vi "Puntje 2 implementeren kladversie.vi"() -> ()   [LabVIEW 2019]
panel:
  in  "Slide 2":dbl(slide) scale=0.0..10.0
  in  "Slide":dbl(slide) scale=0.0..10.0
  out "linkermotor":dbl(knob) scale=0.0..10.0
  out "rechtermotor":dbl(knob) scale=0.0..10.0
  in  "Array":dbl[](array[numeric])
  # "5 : neemt volledig WITTE regio waar"
  # "0 : neemt volledige ZWARTE regio waar"
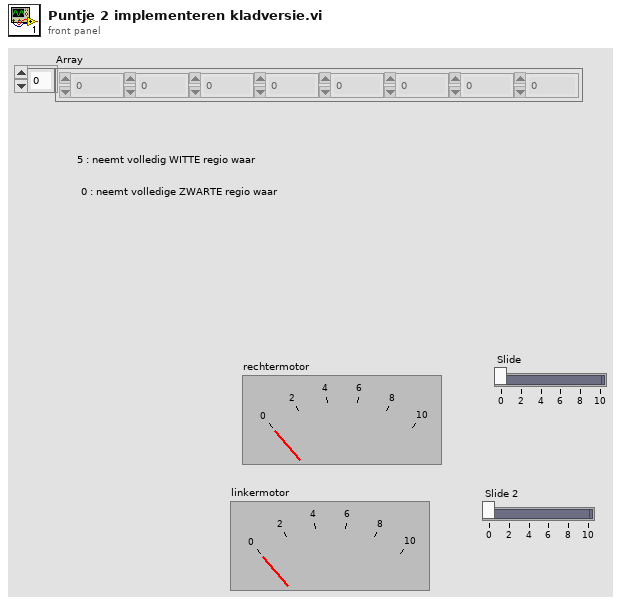
[diagram p1: front panel]
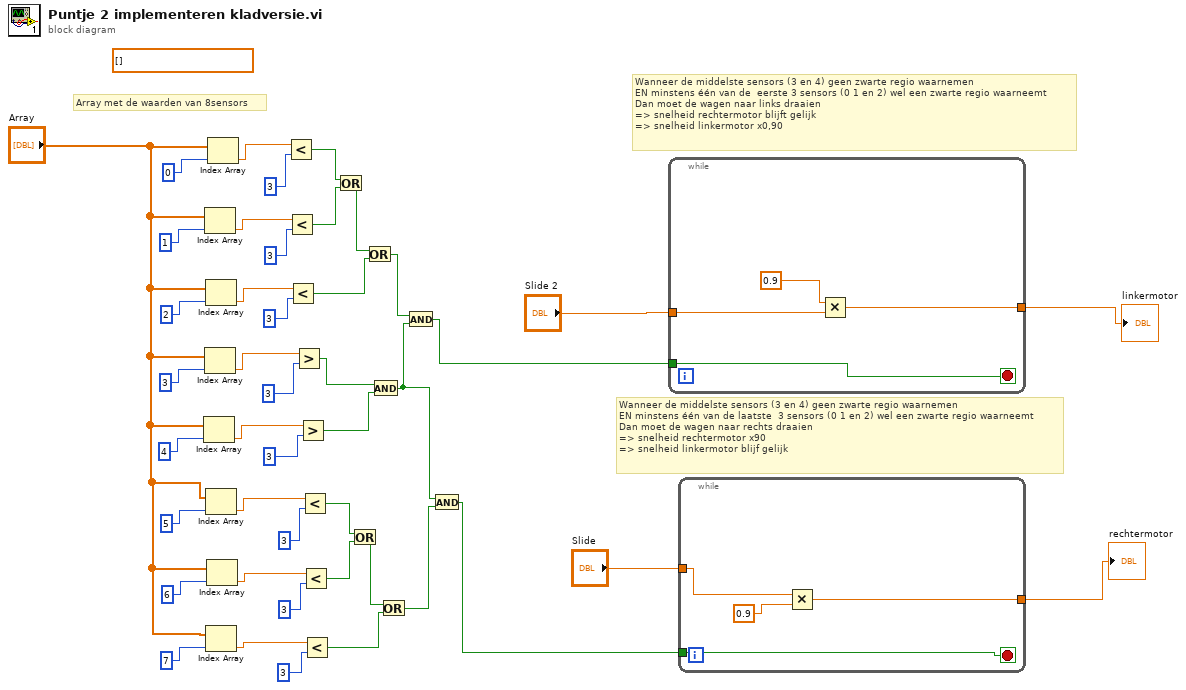
[diagram p0: block diagram]
diagram:
  (unwired) dbl[] []
  # "Wanneer de middelste sensors (3 en 4) geen zwarte regio waarnemen\nEN minstens één van de laatste  3 sensors (0 1 en 2) wel een zwarte regio waarneemt \nDan moet de wagen naar rechts draaien \n=> snelheid rechtermotor x90\n=> snelheid linkermotor blijf gelijk"
  # "Wanneer de middelste sensors (3 en 4) geen zwarte regio waarnemen\nEN minstens één van de  eerste 3 sensors (0 1 en 2) wel een zwarte regio waarneemt \nDan moet de wagen naar links draaien \n=> snelheid rechtermotor blijft gelijk\n=> snelheid linkermotor x0,90"
  # "Array met de waarden van 8sensors"
  n1 = Index Array(array="Array", index=4) -> (element=w35:dbl)
  n2 = Index Array(array="Array", index=1) -> (element=w26:dbl)
  n3 = Index Array(array="Array", index=3) -> (element=w33:dbl)
  n4 = Index Array(array="Array", index=2) -> (element=w28:dbl)
  n5 = Index Array(array="Array", index=5) -> (element=w8:dbl)
  n6 = Index Array(array="Array", index=7) -> (element=w6:dbl)
  n7 = Index Array(array="Array", index=6) -> (element=w7:dbl)
  n8 = Index Array(array="Array", index=0) -> (element=w25:dbl)
  n9 = Less?(x=w25, y=3) -> (x < y?=w23:bool)
  n10 = Less?(x=w26, y=3) -> (x < y?=w22:bool)
  n11 = Less?(x=w28, y=3) -> (x < y?=w20:bool)
  n12 = Greater?(x=w33, y=3) -> (0:w31:bool)
  n13 = Greater?(x=w35, y=3) -> (0:w30:bool)
  n14 = Less?(x=w8, y=3) -> (x < y?=w12:bool)
  n15 = Less?(x=w7, y=3) -> (x < y?=w11:bool)
  n16 = Less?(x=w6, y=3) -> (x < y?=w9:bool)
  n17 = Or(x=w23, y=w22) -> (x .or. y?=w21:bool)
  n18 = Or(x=w12, y=w11) -> (x .or. y?=w10:bool)
  n19 = Or(x=w21, y=w20) -> (x .or. y?=w19:bool)
  n20 = And(x=w31, y=w30) -> (x .and. y?=w5:bool)
  n21 = Or(x=w10, y=w9) -> (x .or. y?=w4:bool)
  n22 = And(x=w19, y=w5) -> (x .and. y?=w18:bool)
  n23 = And(x=w5, y=w4) -> (x .and. y?=w3:bool)
  n24 = while {
    tunnel: w18 -> [w48]
    tunnel: "Slide 2" -> [w47]
    tunnel: [w45] -> w16
    stop <- w48 stop-if-true
    n25 = Multiply(x=0.9, y=w47) -> (x*y=w45:dbl)
  }
  "linkermotor" <- w16
  n26 = while {
    tunnel: w3 -> [w52]
    tunnel: "Slide" -> [w51]
    tunnel: [w49] -> w1
    stop <- w52 stop-if-true
    n27 = Multiply(x=w51, y=0.9) -> (x*y=w49:dbl)
  }
  "rechtermotor" <- w1
